vi "ReadConnInfoUSB.vi"(8 "error in (no error)":errorcluster, 11 "path":path) -> (0 "error out":errorcluster, 2 "found":bool, 3 "connection info":T1={"ClientName"="", "TransceiverHost"="", "TransceiverPort"=6342, "Password"=""})   [LabVIEW 2017, in "USBDrive.lvlib"]
uses:
  <vilib>/addons/InsightCM/Devices/Shared/Common/USBDrive/USBDrive.lvlib
  <vilib>/addons/InsightCM/MessageBus/Base/controls/ConnectionInfo.ctl
  <vilib>/addons/InsightCM/Devices/Shared/Common/ServerComm/ServerComm.lvlib
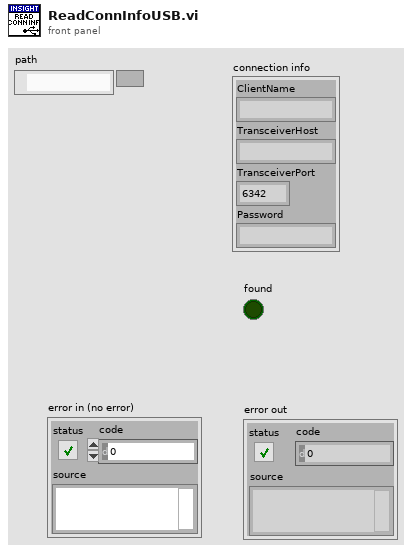
[diagram p1: front panel]
types:
  T1 = typedef "ConnectionInfo.ctl" = cluster{"ClientName":string, "TransceiverHost":string, "TransceiverPort":u16, "Password":string}
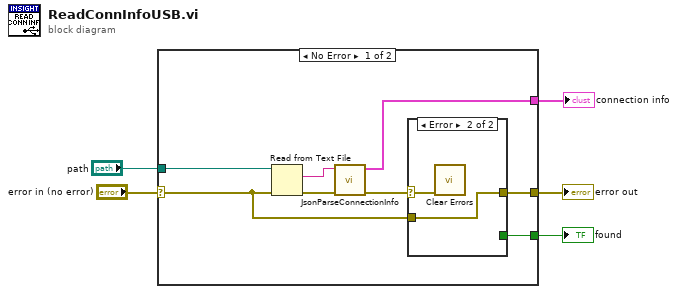
[diagram p0: block diagram]
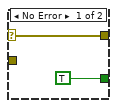
[diagram p2: hidden frame]
diagram:
  n1 = case shown="No Error" "error in (no error)" {
    selector: "error in (no error)" -> [w6 w18]
    tunnel: [w12 w18] -> w4
    tunnel: [w13 _] -> w3
    tunnel: [w10 _] -> w2
    tunnel: "path" -> [w8 _]
    frame No Error {
      n2 = Read from Text File(file (use dialog)=w8, error in=w6) -> (text=w7:string, error out=w9:errorcluster)  [unwired: 2 in, 2 out]
      n3 = call <vilib>:"JsonParseConnectionInfo.vi"("error in (no error)"=w9, "JSON string"=w7) -> ("error out"=w11:errorcluster, "connection info"=w13:T1)  [unwired: 8 in]
      n4 = case shown="Error" w11 {
        selector: w11 -> [w15 w17]
        tunnel: [w15 w16] -> w12
        tunnel: [TRUE _] -> w10
        tunnel: w6 -> [_ w16]
        frame No Error {
        }
        frame Error {
          n5 = call <vilib>:"Clear Errors.vi"("error in (no error)"=w17) -> ()  [unwired: 5 in, 2 out]
        }
      }
    }
    frame Error {
    }
  }
  "error out" <- w4
  "connection info" <- w3
  "found" <- w2
